vi "Read.vi"(8 "error in (no error)":errorcluster, 11 "One Terminal in":refnum<class "AbsFunc_One Term_Bool.lvclass">) -> (0 "error out":errorcluster, 2 "Boolean":bool, 3 "One Terminal out":refnum<class "AbsFunc_One Term_Bool.lvclass">)   [LabVIEW 2021, in "AbsFunc_One Term_Bool.lvclass"]
uses:
  AbsFunc_One Term_Bool.lvclass
  AbsFunc_One Term_Bool.lvclass/AbsFunc_One Term_Bool.ctl
  Abs_Types/Boolean/Abs_Boolean.lvclass
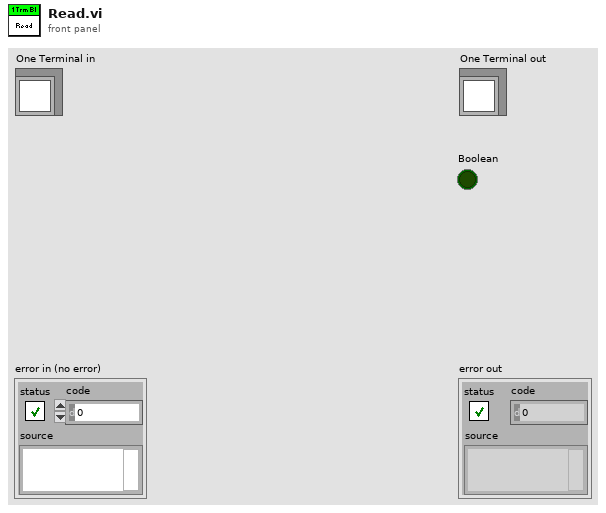
[diagram p1: front panel]
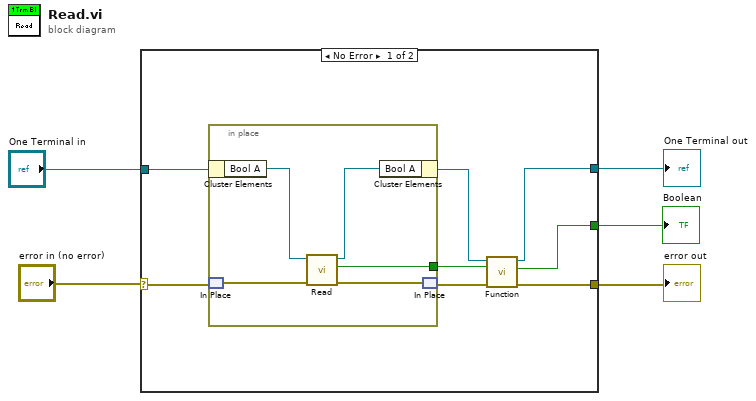
[diagram p0: block diagram]
diagram:
  n1 = case shown="No Error" "error in (no error)" {
    selector: "error in (no error)" -> [w13 w19]
    tunnel: "One Terminal in" -> [w12 w20]
    tunnel: [w8 w20] -> w3
    tunnel: [w7 w19] -> w2
    tunnel: [w6 _] -> w1
    frame No Error {
      n2 = in-place {
        in-place-border: [w14] -> w9
        n3 = in-place-cluster #1(w12) -> ("Bool A"=w18:refnum<class "Abs_Boolean.lvclass">)
        n4 = in-place-match #2(w13) -> (w16:errorcluster)
        n5 = call-dynamic "Read.vi"("error in (no error)"=w16, "Boolean in"=w18) -> ("error out"=w15:errorcluster, "Boolean"=w14:bool, "Boolean out"=w17:refnum<class "Abs_Boolean.lvclass">)  [unwired: 7 in]
        n6 = in-place-cluster #1("Bool A"=w17) -> (w10:refnum<class "AbsFunc_One Term_Bool.lvclass">)
        n7 = in-place-match #2(w15) -> (w11:errorcluster)
      }
      n8 = call-dynamic "Function.vi"("error in (no error)"=w11, "Boolean A"=w9, "One Terminal in"=w10) -> ("error out"=w7:errorcluster, "Boolean"=w6:bool, "One Terminal out"=w8:refnum<class "AbsFunc_One Term_Bool.lvclass">)  [unwired: 6 in]
    }
    frame Error {
    }
  }
  "error out" <- w2
  "One Terminal out" <- w3
  "Boolean" <- w1
